vi "StateHapticEngine.vi"(0 "Master State In":T1(ring)) -> ()   [LabVIEW 2023]
doc: "Manages the haptic feedback on the driver and manipulator joysticks."
uses:
  GlobalDriverStationData.vi
  GlobalAutonomous.vi
  GlobalDriverStationCommands.vi
  GRNF_Joystick.vi
  GlobalDrivebase.vi
  GlobalNoteHandling.vi
panel:
  in  "Develop New Haptic":bool
  in  "Duty Cycle (%)":dbl=100.0
  in  "Amplitude":dbl=1.0
  in  "Period (s)":dbl=10.0
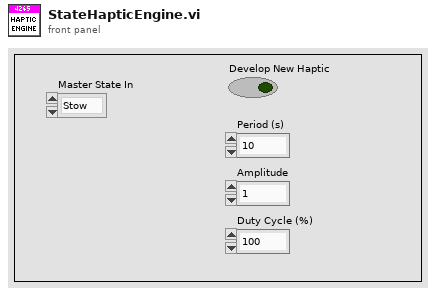
[diagram p1: front panel]
types:
  T1 = enum16{"Stow", "Speaker", "Amp", "Climbing", "Trap"}
  T2 = enum16{"None", "Development", "Longpress Buttons", "Intaking"}
  T3 = typedef "WPI_JoystickDevRef.ctl" = cluster{"Device":T4}
  T4 = typedef "WPI_JoystickDeviceEnum.ctl" = enum16{"USB 0", "USB 1", "USB 2", "USB 3", "USB 4", "USB 5"}
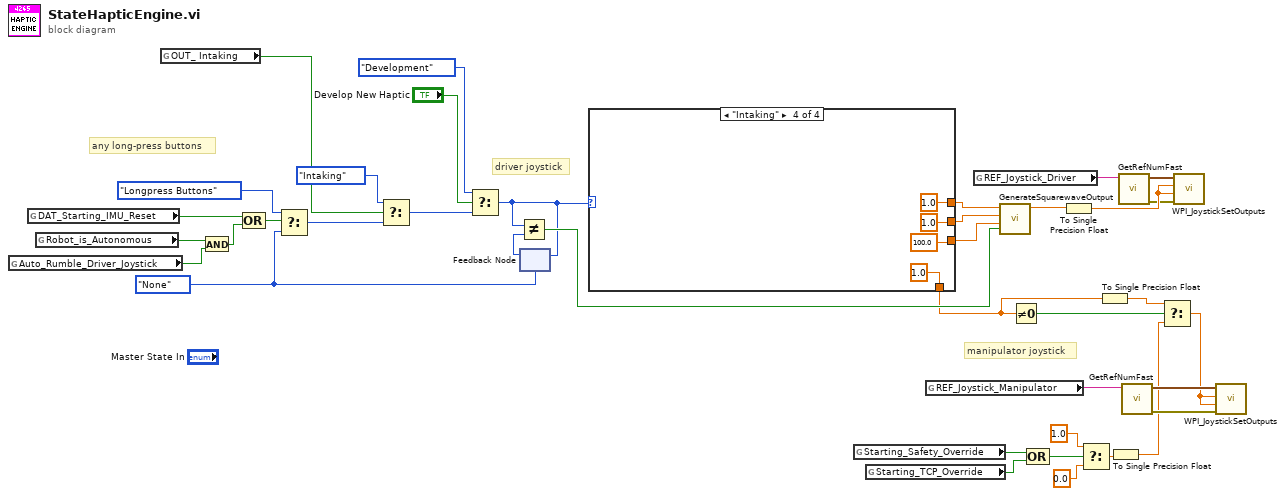
[diagram p0: block diagram]
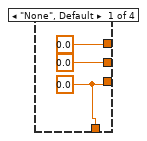
[diagram p2: hidden frame]
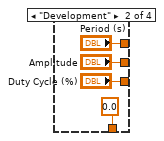
[diagram p3: hidden frame]
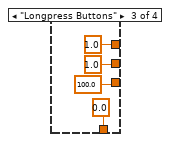
[diagram p4: hidden frame]
diagram:
  w9 = T2."None"
  # "any long-press buttons"
  # "manipulator joystick"
  # "driver joystick"
  n1 = global read "GlobalAutonomous.vi" "Auto_Rumble_Driver_Joystick"() -> (w28:bool)
  n2 = global read "GlobalDrivebase.vi" "DAT_Starting_IMU_Reset"() -> (w12:bool)
  n3 = global read "GlobalDriverStationData.vi" "Robot_is_Autonomous"() -> (w17:bool)
  n4 = global read "GlobalNoteHandling.vi" "OUT_ Intaking"() -> (w7:bool)
  n5 = And(x=w17, y=w28) -> (x .and. y?=w27:bool)
  n6 = Compound Arithmetic op=OR(w12, w27) -> (w25:bool)
  n7 = Select(t=T2."Longpress Buttons", s=w25, f=w9) -> (s? t:f=w15:T2)
  n8 = Select(t=T2."Intaking", s=w7, f=w15) -> (s? t:f=w8:T2)
  n9 = Select(t=T2."Development", s="Develop New Haptic", f=w8) -> (s? t:f=w21:T2)
  n10 = feedback-in #1(w21) -> ()
  n11 = feedback #1(w9) -> (w24:T2)
  n12 = Not Equal?(x=w21, y=w24) -> (x != y?=w23:bool)
  n13 = case shown="\"Intaking\"" w21 {
    tunnel: [0.0 ("Period (s)") "Period (s)" 1.0 ("Period (s)") 1.0 ("Period (s)")] -> w20
    tunnel: [0.0 ("Amplitude") "Amplitude" 1.0 ("Amplitude") 1.0 ("Amplitude")] -> w19
    tunnel: [w39 "Duty Cycle (%)" 100.0 ("Duty Cycle (%)") 100.0 ("Duty Cycle (%)")] -> w18
    tunnel: [w39 0.0 ("Period (s)") 0.0 ("Period (s)") 1.0 ("Period (s)")] -> w2
    frame "None", Default {
      w39 = 0.0 ("Duty Cycle (%)")
    }
    frame "Development" {
    }
    frame "Longpress Buttons" {
    }
    frame "Intaking" {
    }
  }
  n14 = global read "GlobalDriverStationData.vi" "Starting_Safety_Override"() -> (w29:bool)
  n15 = global read "GlobalDriverStationData.vi" "Starting_TCP_Override"() -> (w16:bool)
  n16 = global read "GlobalDriverStationCommands.vi" "REF_Joystick_Manipulator"() -> (w14:string)
  n17 = global read "GlobalDriverStationCommands.vi" "REF_Joystick_Driver"() -> (w13:string)
  n18 = call "GenerateSquarewaveOutput.vi"("Init"=w23, "Duty Cycle (%)"=w18, "Amplitude"=w19, "Period (s)"=w20) -> ("Square Wave Ouput"=w26:dbl)  [unwired: 7 in]
  n19 = Not Equal To 0?(x=w2) -> (x != 0?=w5:bool)
  n20 = Compound Arithmetic op=OR(w29, w16) -> (w34:bool)
  n21 = To Single Precision Float(number=w26) -> (single precision float=w38:sgl)
  n22 = Select(t=1.0, s=w34, f=0.0) -> (s? t:f=w35:dbl)
  n23 = To Single Precision Float(number=w2) -> (single precision float=w1:sgl)
  n24 = To Single Precision Float(number=w35) -> (single precision float=w4:sgl)
  n25 = call-poly "GetRefNumFast.vi"("RefNum Name"=w13) -> ("Error"=w32:errorcluster, "Device Reference"=w33:T3)  [unwired: 5 in]
  n26 = call-poly "GetRefNumFast.vi"("RefNum Name"=w14) -> ("Error"=w31:errorcluster, "Device Reference"=w30:T3)  [unwired: 5 in]
  n27 = Select(t=w1, s=w5, f=w4) -> (s? t:f=w3:sgl)
  n28 = call <vilib>:"WPI_JoystickSetOutputs.vi"("error in (no error)"=w32, "Right Rumble"=w38, "Left Rumble"=w38, "JoystickDevRef"=w33) -> ()  [unwired: 6 in, 2 out]
  n29 = call <vilib>:"WPI_JoystickSetOutputs.vi"("error in (no error)"=w31, "Right Rumble"=w3, "Left Rumble"=w3, "JoystickDevRef"=w30) -> ()  [unwired: 6 in, 2 out]
